vi "メイン.vi"() -> (2 "測定周期/ms":dbl, 3 "値転記用配列":T2[](array[typedef]))   [LabVIEW 2021] (continued)
                            n1019 = call-poly <vilib>:"Read Key.vi"("section"=w2857, "error in (no error)"=w2856, "key"=w2853, "refnum"=w2859) -> ("error out"=w2855:errorcluster, "value"=w2854:i32, "refnum out"=w2858:T10)  [unwired: 4 in, 1 out]
                            n1020 = Bundle By Name(cluster=w2851, "ポートNo."=w2854) -> (w2852:T2)
                          }
                          frame 4 {
                            n1021 = call-poly <vilib>:"Read Key.vi"("section"=w2866, "error in (no error)"=w2865, "key"=w2862, "refnum"=w2868) -> ("error out"=w2864:errorcluster, "value"=w2863:i32, "refnum out"=w2867:T10)  [unwired: 4 in, 1 out]
                            n1022 = Bundle By Name(cluster=w2860, "測定モード"=w2863) -> (w2861:T2)
                          }
                          frame 5 {
                            n1023 = call-poly <vilib>:"Read Key.vi"("section"=w2875, "error in (no error)"=w2874, "key"=w2871, "refnum"=w2877) -> ("error out"=w2873:errorcluster, "value"=w2872:string, "refnum out"=w2876:T10)  [unwired: 4 in, 1 out]
                            n1024 = Bundle By Name(cluster=w2870, "規格単位"=w2872) -> (w2869:T2)
                          }
                          frame 6 {
                            n1025 = call-poly <vilib>:"Read Key.vi"("section"=w2884, "error in (no error)"=w2883, "key"=w2880, "refnum"=w2886) -> ("error out"=w2882:errorcluster, "value"=w2881:string, "refnum out"=w2885:T10)  [unwired: 4 in, 1 out]
                            n1026 = Bundle By Name(cluster=w2879, "品質チェック項目"=w2881) -> (w2878:T2)
                          }
                          frame 7 {
                            n1027 = call-poly <vilib>:"Read Key.vi"("section"=w2893, "error in (no error)"=w2892, "key"=w2889, "refnum"=w2895) -> ("error out"=w2891:errorcluster, "value"=w2890:i32, "refnum out"=w2894:T10)  [unwired: 4 in, 1 out]
                            n1028 = Bundle By Name(cluster=w2888, "測定周期"=w2890) -> (w2887:T2)
                          }
                          frame 8 {
                            n1029 = call-poly <vilib>:"Read Key.vi"("section"=w2902, "error in (no error)"=w2901, "key"=w2898, "refnum"=w2904) -> ("error out"=w2900:errorcluster, "value"=w2899:string, "refnum out"=w2903:T10)  [unwired: 4 in, 1 out]
                            n1030 = Bundle By Name(cluster=w2896, "実測値MAX"=w2899) -> (w2897:T2)
                          }
                          frame 9 {
                            n1031 = call-poly <vilib>:"Read Key.vi"("section"=w2911, "error in (no error)"=w2910, "key"=w2907, "refnum"=w2913) -> ("error out"=w2909:errorcluster, "value"=w2908:string, "refnum out"=w2912:T10)  [unwired: 4 in, 1 out]
                            n1032 = Bundle By Name(cluster=w2905, "実測値MIN"=w2908) -> (w2906:T2)
                          }
                          frame 10 {
                            n1033 = call-poly <vilib>:"Read Key.vi"("section"=w2920, "error in (no error)"=w2919, "key"=w2916, "refnum"=w2922) -> ("error out"=w2918:errorcluster, "value"=w2917:string, "refnum out"=w2921:T10)  [unwired: 4 in, 1 out]
                            n1034 = Bundle By Name(cluster=w2914, "実測値(MAX)"=w2917) -> (w2915:T2)
                          }
                          frame 11 {
                            n1035 = call-poly <vilib>:"Read Key.vi"("section"=w2929, "error in (no error)"=w2928, "key"=w2925, "refnum"=w2931) -> ("error out"=w2927:errorcluster, "value"=w2926:string, "refnum out"=w2930:T10)  [unwired: 4 in, 1 out]
                            n1036 = Bundle By Name(cluster=w2923, "実測値(MIN)"=w2926) -> (w2924:T2)
                          }
                          frame 12 {
                            n1037 = call-poly <vilib>:"Read Key.vi"("section"=w2938, "error in (no error)"=w2937, "key"=w2934, "refnum"=w2940) -> ("error out"=w2936:errorcluster, "value"=w2935:bool, "refnum out"=w2939:T10)  [unwired: 4 in, 1 out]
                            n1038 = Bundle By Name(cluster=w2932, "測定画面表示ボタン"=w2935) -> (w2933:T2)
                          }
                          frame 13 {
                            n1039 = call-poly <vilib>:"Read Key.vi"("section"=w2947, "error in (no error)"=w2946, "key"=w2943, "refnum"=w2949) -> ("error out"=w2945:errorcluster, "value"=w2944:string, "refnum out"=w2948:T10)  [unwired: 4 in, 1 out]
                            n1040 = Bundle By Name(cluster=w2941, "ゲージポートNo"=w2944) -> (w2942:T2)
                          }
                        }
                        n1041 = local write "メイン設定_設定 12"(w2817) -> ()
                      }
                      n1042 = local read "メインON/OFF_\n設定 12"() -> (w2801:T1)
                      n1043 = call-poly <vilib>:"Read Key.vi"("section"=w2790, "error in (no error)"=w2808, "key"="使用ON/OFF", "refnum"=w2809) -> ("error out"=w2793:errorcluster, "value"=w2799:bool, "refnum out"=w2794:T10)  [unwired: 4 in, 1 out]
                      n1044 = Bundle By Name(cluster=w2801, "使用ON/OFF"=w2799) -> (w2802:T1)
                      n1045 = local write "メインON/OFF_\n設定 12"(w2802) -> ()
                      n1046 = local read "CSV項目名 12"() -> (w2798:T3)
                      n1047 = call-poly <vilib>:"Read Key.vi"("section"=w2790, "error in (no error)"=w2793, "key"="CSVヘッダー名", "refnum"=w2794) -> ("error out"=w2791:errorcluster, "value"=w2796:string, "refnum out"=w2792:T10)  [unwired: 4 in, 1 out]
                      n1048 = Bundle By Name(cluster=w2798, "CSV項目名"=w2796) -> (w2797:T3)
                      n1049 = local write "CSV項目名 12"(w2797) -> ()
                    }
                    frame #1 {
                      # "csvヘッダー項目作成"
                      # "⑮"
                      # "⑤"
                      n1050 = local read "CSV項目名 12"() -> (w2954:T3)
                      n1051 = Unbundle By Name(w2954) -> ("CSV項目名"=w2951:string)
                      n1052 = local read "メイン設定_設定 12"() -> (w2955:T2)
                      n1053 = Unbundle By Name(w2955) -> ("測定モード"=w2950:u16)
                      n1054 = case shown="0, デフォルト" w2950 {
                        tunnel: ["単発測定" _ "多点測定"] -> w2958
                        tunnel: [FALSE TRUE FALSE] -> w2957
                        tunnel: [TRUE FALSE TRUE] -> w2956
                        frame 0, Default {
                        }
                        frame 1 {
                        }
                        frame 2 {
                        }
                      }
                      n1055 = case shown="1" w2950 {
                        tunnel: w2951 -> [w2964 w2976 w2985]
                        tunnel: [w2962 w2974 w2987] -> w2953
                        tunnel: [w2961 w2973 w2986] -> w2952
                        frame 1 {
                          n1056 = Empty String/Path?(string/path=w2964) -> (empty?=w2963:bool)
                          n1057 = case shown="FALSE" w2963 {
                            tunnel: w2964 -> [w2970 _]
                            tunnel: w2964 -> [w2969 _]
                            tunnel: [w2966 ""] -> w2962
                            tunnel: [w2965 ""] -> w2961
                            frame False {
                              n1058 = Concatenate Strings(w2970, "_max") -> (w2966:string)
                              n1059 = Concatenate Strings(w2969, "_min") -> (w2965:string)
                            }
                            frame True {
                            }
                          }
                        }
                        frame 2 {
                          n1060 = Empty String/Path?(string/path=w2976) -> (empty?=w2975:bool)
                          n1061 = case shown="FALSE" w2975 {
                            tunnel: w2976 -> [w2982 _]
                            tunnel: w2976 -> [w2981 _]
                            tunnel: [w2978 ""] -> w2974
                            tunnel: [w2977 ""] -> w2973
                            frame False {
                              n1062 = Concatenate Strings(w2982, "_max") -> (w2978:string)
                              n1063 = Concatenate Strings(w2981, "_min") -> (w2977:string)
                            }
                            frame True {
                            }
                          }
                        }
                        frame 0, Default {
                          n1064 = Empty String/Path?(string/path=w2985) -> (empty?=w2988:bool)
                          n1065 = case shown="FALSE" w2988 {
                            tunnel: w2985 -> [w2992 _]
                            tunnel: [w2990 ""] -> w2987
                            tunnel: ["" ""] -> w2986
                            frame False {
                              n1066 = Concatenate Strings(w2992, "_value") -> (w2990:string)
                            }
                            frame True {
                            }
                          }
                        }
                      }
                      n1067 = property on="メイン測定ボタン_単発 12" class="Bool (指定)"("BoolText.Text"=w2958) -> ()  [unwired: 2 in, 2 out]
                      n1068 = local write "csv入力項目min 12"(w2952) -> ()
                      n1069 = local write "csv入力項目max 12"(w2953) -> ()
                      n1070 = property on="メイン測定ボタン_連続 12" class="Bool (指定)"("Visible"=w2957) -> ()  [unwired: 2 in, 2 out]
                      n1071 = property on="メイン測定ボタン_単発 12" class="Bool (指定)"("Visible"=w2956) -> ()  [unwired: 2 in, 2 out]
                    }
                    frame #2 {
                      # "⑯"
                      # "⑨"
                      # "⑧"
                      # "⑦"
                      # "⑥"
                      n1072 = local read "メインON/OFF_\n設定 12"() -> (w3006:T1)
                      n1073 = local write "メインON/OFF_\n保存確認 12"(w3006) -> ()
                      n1074 = local read "メイン設定_設定 12"() -> (w3004:T2)
                      n1075 = Unbundle By Name(w3004) -> ("測定画面表示ボタン"=w3003:bool)
                      n1076 = case shown="FALSE" w3003 {
                        tunnel: [w3009 TRUE] -> w3005
                        frame False {
                          w3009 = FALSE
                          n1077 = property on="メイン測定ボタン_単発 12" class="Bool (指定)"("Visible"=w3009) -> ()  [unwired: 2 in, 2 out]
                          n1078 = property on="メイン測定ボタン_連続 12" class="Bool (指定)"("Visible"=w3009) -> ()  [unwired: 2 in, 2 out]
                        }
                        frame True {
                        }
                      }
                      n1079 = local write "メインON/OFF_制御器 12"(w3006) -> ()
                      n1080 = property on="メインON/OFF_制御器 12" class="Clust (指定)"("Visible"=w3005) -> ()  [unwired: 2 in, 2 out]
                      n1081 = property on="メイン設定No_設定 12" class="Clust (指定)"("Visible"=w3005) -> ()  [unwired: 2 in, 2 out]
                      n1082 = property on="メイン設定_設定 12" class="Clust (指定)"("Visible"=w3005) -> ()  [unwired: 2 in, 2 out]
                      n1083 = property on="キャンセルボタン 12" class="Bool (指定)"("Visible"=w3005) -> ()  [unwired: 2 in, 2 out]
                    }
                  }
                  n1084 = Replace Array Subset(array=w2785, new element=w2777, index=11) -> (w2784:T2[])
                }
              }
              n1085 = property on="値転記用配列" class="Arr (指定)"("Value"=w70) -> ()  [unwired: 2 in, 2 out]
              n1086 = call <vilib>:"Close Config Data.vi"("error in (no error)"=w72, "refnum"=w73) -> ("error out"=→"setup.iniエラーout":errorcluster)  [unwired: 1 in, 8 out]
            }
          }
          frame #1 {
            # "csv作成表　を置換処理させる為の初期化"
            # "csv作成表_csv書込み　を置換処理させる為の初期化"
            n1087 = for {
              N: 3 -> [_]
              tunnel: [w3019] -> w3011 mode=indexing
              i -> [w3020]
              n1088 = case shown="0, デフォルト" w3020 {
                tunnel: [w3021 w3051 w3053] -> w3019
                frame 0, Default {
                  # "CSVマスターインポートファイル名を作成しA1セルに表示"
                  n1089 = local read "CSV保存名"() -> (w3022:string)
                  n1090 = Concatenate Strings("Sokutei_", w3022) -> (w3023:string)
                  n1091 = Build Array(w3023) -> (w3021:string[])
                }
                frame 1 {
                  n1092 = local read "csv入力項目max 11"() -> (w3028:string)
                  n1093 = local read "csv入力項目max 1"() -> (w3048:string)
                  n1094 = local read "csv入力項目max 3"() -> (w3044:string)
                  n1095 = local read "csv入力項目max 5"() -> (w3040:string)
                  n1096 = local read "csv入力項目max 7"() -> (w3036:string)
                  n1097 = local read "csv入力項目max 9"() -> (w3032:string)
                  n1098 = local read "csv入力項目min 11"() -> (w3027:string)
                  n1099 = local read "csv入力項目min 1"() -> (w3047:string)
                  n1100 = local read "csv入力項目min 3"() -> (w3043:string)
                  n1101 = local read "csv入力項目min 5"() -> (w3039:string)
                  n1102 = local read "csv入力項目min 7"() -> (w3035:string)
                  n1103 = local read "csv入力項目min 9"() -> (w3031:string)
                  n1104 = local read "csv入力項目max 2"() -> (w3046:string)
                  n1105 = local read "csv入力項目max 4"() -> (w3042:string)
                  n1106 = local read "csv入力項目max 6"() -> (w3038:string)
                  n1107 = local read "csv入力項目max 8"() -> (w3034:string)
                  n1108 = local read "csv入力項目max 10"() -> (w3030:string)
                  n1109 = local read "csv入力項目max 12"() -> (w3026:string)
                  n1110 = local read "csv入力項目min 2"() -> (w3045:string)
                  n1111 = local read "csv入力項目min 4"() -> (w3041:string)
                  n1112 = local read "csv入力項目min 6"() -> (w3037:string)
                  n1113 = local read "csv入力項目min 8"() -> (w3033:string)
                  n1114 = local read "csv入力項目min 10"() -> (w3029:string)
                  n1115 = local read "csv入力項目min 12"() -> (w3025:string)
                  n1116 = Build Array("Date", "Time", w3048, w3047, w3046, w3045, w3044, w3043, w3042, w3041, w3040, w3039, w3038, w3037, w3036, w3035, w3034, w3033, w3032, w3031, w3030, w3029, w3028, w3027, w3026, w3025) -> (w3051:string[])
                }
                frame 2 {
                  # "csv作成表の3行目の初期化\n配列置換する為の処理　\n並列処理は仮\nループ使用で考え直す"
                  n1117 = call <vilib>:"Space Constant.vi"() -> ("String"=w3052:string)
                  n1118 = Build Array(w3052, w3052, w3052, w3052, w3052, w3052, w3052, w3052, w3052, w3052, w3052, w3052, w3052, w3052, w3052, w3052, w3052, w3052, w3052, w3052, w3052, w3052, w3052, w3052, w3052, w3052, w3052, w3052, w3052, w3052, w3052, w3052, w3052, w3052, w3052, w3052, w3052, w3052, w3052, w3052, w3052, w3052, w3052, w3052, w3052) -> (w3053:string[])
                }
              }
            }
            n1119 = for {
              N: 66 -> [_]
              i -> [w3017]
              n1120 = local read "csv作成表_csv書込"() -> (w3018:string[][])
              n1121 = Insert Into Array(array=w3018, index (col)=w3017, new element=string[][] [["  ", " ", " "], ["  ", "", ""], ["  ", "", ""]]) -> (w3015:string[][])  [unwired: 1 in]
              n1122 = local write "csv作成表_csv書込_リセット用"(w3015) -> ()
              n1123 = local write "csv作成表_csv書込"(w3015) -> ()
            }
            n1124 = local write "csv作成表_リセット用"(w3011) -> ()
            n1125 = local write "csv作成表"(w3011) -> ()
          }
        }
      }
      frame "ON/OFF1" {
        # "①"
        # "②"
        # "他複製時に変更する項目\n①②\nローカル変数"
        # "メイン画面で作業者が測定値の転記のON/OFFを設定する"
        n1126 = local read "メインON/OFF_制御器 1"() -> (w3054:T1)
        n1127 = local write "メインON/OFF_\n設定 1"(w3054) -> ()
      }
      frame "ON/OFF2" {
        # "①"
        # "②"
        # "他複製時に変更する項目\n①②\nローカル変数"
        # "メイン画面で作業者が測定値の転記のON/OFFを設定する"
        n1128 = local read "メインON/OFF_制御器 2"() -> (w3056:T1)
        n1129 = local write "メインON/OFF_\n設定 2"(w3056) -> ()
      }
      frame "ON/OFF3" {
        # "①"
        # "②"
        # "他複製時に変更する項目\n①②\nローカル変数"
        # "メイン画面で作業者が測定値の転記のON/OFFを設定する"
        n1130 = local read "メインON/OFF_制御器 3"() -> (w3058:T1)
        n1131 = local write "メインON/OFF_\n設定 3"(w3058) -> ()
      }
      frame "ON/OFF4" {
        # "①"
        # "②"
        # "他複製時に変更する項目\n①②\nローカル変数"
        # "メイン画面で作業者が測定値の転記のON/OFFを設定する"
        n1132 = local read "メインON/OFF_制御器 4"() -> (w3060:T1)
        n1133 = local write "メインON/OFF_\n設定 4"(w3060) -> ()
      }
      frame "ON/OFF5" {
        # "①"
        # "②"
        # "他複製時に変更する項目\n①②\nローカル変数"
        # "メイン画面で作業者が測定値の転記のON/OFFを設定する"
        n1134 = local read "メインON/OFF_制御器 5"() -> (w3062:T1)
        n1135 = local write "メインON/OFF_\n設定 5"(w3062) -> ()
      }
      frame "ON/OFF6" {
        # "①"
        # "②"
        # "他複製時に変更する項目\n①②\nローカル変数"
        # "メイン画面で作業者が測定値の転記のON/OFFを設定する"
        n1136 = local read "メインON/OFF_制御器 6"() -> (w3064:T1)
        n1137 = local write "メインON/OFF_\n設定 6"(w3064) -> ()
      }
      frame "ON/OFF7" {
        # "①"
        # "②"
        # "他複製時に変更する項目\n①②\nローカル変数"
        # "メイン画面で作業者が測定値の転記のON/OFFを設定する"
        n1138 = local read "メインON/OFF_制御器 7"() -> (w3066:T1)
        n1139 = local write "メインON/OFF_\n設定 7"(w3066) -> ()
      }
      frame "ON/OFF8" {
        # "①"
        # "②"
        # "他複製時に変更する項目\n①②\nローカル変数"
        # "メイン画面で作業者が測定値の転記のON/OFFを設定する"
        n1140 = local read "メインON/OFF_制御器 8"() -> (w3068:T1)
        n1141 = local write "メインON/OFF_\n設定 8"(w3068) -> ()
      }
      frame "ON/OFF9" {
        # "①"
        # "②"
        # "他複製時に変更する項目\n①②\nローカル変数"
        # "メイン画面で作業者が測定値の転記のON/OFFを設定する"
        n1142 = local read "メインON/OFF_制御器 9"() -> (w3070:T1)
        n1143 = local write "メインON/OFF_\n設定 9"(w3070) -> ()
      }
      frame "ON/OFF10" {
        # "①"
        # "②"
        # "他複製時に変更する項目\n①②\nローカル変数"
        # "メイン画面で作業者が測定値の転記のON/OFFを設定する"
        n1144 = local read "メインON/OFF_制御器 10"() -> (w3072:T1)
        n1145 = local write "メインON/OFF_\n設定 10"(w3072) -> ()
      }
      frame "ON/OFF11" {
        # "①"
        # "②"
        # "他複製時に変更する項目\n①②\nローカル変数"
        # "メイン画面で作業者が測定値の転記のON/OFFを設定する"
        n1146 = local read "メインON/OFF_制御器 11"() -> (w3074:T1)
        n1147 = local write "メインON/OFF_\n設定 11"(w3074) -> ()
      }
      frame "ON/OFF12" {
        # "①"
        # "②"
        # "他複製時に変更する項目\n①②\nローカル変数"
        # "メイン画面で作業者が測定値の転記のON/OFFを設定する"
        n1148 = local read "メインON/OFF_制御器 12"() -> (w3076:T1)
        n1149 = local write "メインON/OFF_\n設定 12"(w3076) -> ()
      }
      frame "TOPページへ" {
        w3078 = TRUE
        # "メインviを閉じるのみの動作"
        n1150 = flat-sequence {
          tunnel: w3078 -> [w3080]
          tunnel: [w3081] -> w3079
          tunnel: w3078 -> [w3081]
          frame #0 {
            n1151 = global write "VISA停止_G.vi" "VISA停止_\nグローバル"(w3080) -> ()
          }
          frame #1 {
          }
        }
      }
      frame "保存せず" {
        w3087 = T9 {"Horizontal"=-51, "Vertical"=0} ("座標 1")
        # "csv作成表の初期化"
        # "赤枠の初期化"
        # "②"
        # "①"
        # "全ての項目に適応の為、このケースでのみで処理"
        # "①測定値を空にする処理\n複製した項目を追加する必要がある\n②測定新値リセットをFalseにする\nⅠ.初期設定⑥\nと同じなので、どちらか項目を追加したらコピーする"
        n1152 = for {
          N: 32 -> [_]
          i -> [w3106]
          n1153 = case shown="0, デフォルト" w3106 {
            frame 0, Default {
              w3109 = ""
              n1154 = local read "メイン設定_設定 1"() -> (w3108:T2)
              n1155 = Bundle By Name(cluster=w3108, "実測値(MAX)"=w3109, "実測値(MIN)"=w3109) -> (w3107:T2)
              n1156 = local write "メイン設定_設定 1"(w3107) -> ()
            }
            frame 1 {
              w3112 = ""
              n1157 = local read "メイン設定_設定 2"() -> (w3111:T2)
              n1158 = Bundle By Name(cluster=w3111, "実測値(MAX)"=w3112, "実測値(MIN)"=w3112) -> (w3110:T2)
              n1159 = local write "メイン設定_設定 2"(w3110) -> ()
            }
            frame 2 {
              w3115 = ""
              n1160 = local read "メイン設定_設定 3"() -> (w3114:T2)
              n1161 = Bundle By Name(cluster=w3114, "実測値(MAX)"=w3115, "実測値(MIN)"=w3115) -> (w3113:T2)
              n1162 = local write "メイン設定_設定 3"(w3113) -> ()
            }
            frame 3 {
              w3118 = ""
              n1163 = local read "メイン設定_設定 4"() -> (w3117:T2)
              n1164 = Bundle By Name(cluster=w3117, "実測値(MAX)"=w3118, "実測値(MIN)"=w3118) -> (w3116:T2)
              n1165 = local write "メイン設定_設定 4"(w3116) -> ()
            }
            frame 4 {
              w3121 = ""
              n1166 = local read "メイン設定_設定 5"() -> (w3120:T2)
              n1167 = Bundle By Name(cluster=w3120, "実測値(MAX)"=w3121, "実測値(MIN)"=w3121) -> (w3119:T2)
              n1168 = local write "メイン設定_設定 5"(w3119) -> ()
            }
            frame 5 {
              w3124 = ""
              n1169 = local read "メイン設定_設定 6"() -> (w3123:T2)
              n1170 = Bundle By Name(cluster=w3123, "実測値(MAX)"=w3124, "実測値(MIN)"=w3124) -> (w3122:T2)
              n1171 = local write "メイン設定_設定 6"(w3122) -> ()
            }
            frame 6 {
              w3127 = ""
              n1172 = local read "メイン設定_設定 7"() -> (w3126:T2)
              n1173 = Bundle By Name(cluster=w3126, "実測値(MAX)"=w3127, "実測値(MIN)"=w3127) -> (w3125:T2)
              n1174 = local write "メイン設定_設定 7"(w3125) -> ()
            }
            frame 7 {
              w3130 = ""
              n1175 = local read "メイン設定_設定 8"() -> (w3129:T2)
              n1176 = Bundle By Name(cluster=w3129, "実測値(MAX)"=w3130, "実測値(MIN)"=w3130) -> (w3128:T2)
              n1177 = local write "メイン設定_設定 8"(w3128) -> ()
            }
            frame 8 {
              w3133 = ""
              n1178 = local read "メイン設定_設定 9"() -> (w3132:T2)
              n1179 = Bundle By Name(cluster=w3132, "実測値(MAX)"=w3133, "実測値(MIN)"=w3133) -> (w3131:T2)
              n1180 = local write "メイン設定_設定 9"(w3131) -> ()
            }
            frame 9 {
              w3136 = ""
              n1181 = local read "メイン設定_設定 10"() -> (w3135:T2)
              n1182 = Bundle By Name(cluster=w3135, "実測値(MAX)"=w3136, "実測値(MIN)"=w3136) -> (w3134:T2)
              n1183 = local write "メイン設定_設定 10"(w3134) -> ()
            }
            frame 10 {
              w3139 = ""
              n1184 = local read "メイン設定_設定 11"() -> (w3138:T2)
              n1185 = Bundle By Name(cluster=w3138, "実測値(MAX)"=w3139, "実測値(MIN)"=w3139) -> (w3137:T2)
              n1186 = local write "メイン設定_設定 11"(w3137) -> ()
            }
            frame 11 {
              w3142 = ""
              n1187 = local read "メイン設定_設定 12"() -> (w3141:T2)
              n1188 = Bundle By Name(cluster=w3141, "実測値(MAX)"=w3142, "実測値(MIN)"=w3142) -> (w3140:T2)
              n1189 = local write "メイン設定_設定 12"(w3140) -> ()
            }
          }
        }
        n1190 = for {
          N: 32 -> [_]
          tunnel: FALSE -> [w3092]
          i -> [w3093]
          n1191 = case shown="0, デフォルト" w3093 {
            tunnel: w3092 -> [w3094 w3095 w3096 w3097 w3098 w3099 w3100 w3101 w3102 w3103 w3104 w3105]
            frame 0, Default {
              n1192 = local write "測定新値\nリセット用 1"(w3094) -> ()
              n1193 = local write "測定旧値 1"(w3094) -> ()
            }
            frame 1 {
              n1194 = local write "測定新値\nリセット用 2"(w3095) -> ()
              n1195 = local write "測定旧値 2"(w3095) -> ()
            }
            frame 2 {
              n1196 = local write "測定新値\nリセット用 3"(w3096) -> ()
              n1197 = local write "測定旧値 3"(w3096) -> ()
            }
            frame 3 {
              n1198 = local write "測定新値\nリセット用 4"(w3097) -> ()
              n1199 = local write "測定旧値 4"(w3097) -> ()
            }
            frame 4 {
              n1200 = local write "測定新値\nリセット用 5"(w3098) -> ()
              n1201 = local write "測定旧値 5"(w3098) -> ()
            }
            frame 5 {
              n1202 = local write "測定新値\nリセット用 6"(w3099) -> ()
              n1203 = local write "測定旧値 6"(w3099) -> ()
            }
            frame 6 {
              n1204 = local write "測定新値\nリセット用 7"(w3100) -> ()
              n1205 = local write "測定旧値 7"(w3100) -> ()
            }
            frame 7 {
              n1206 = local write "測定新値\nリセット用 8"(w3101) -> ()
              n1207 = local write "測定旧値 8"(w3101) -> ()
            }
            frame 8 {
              n1208 = local write "測定新値\nリセット用 9"(w3102) -> ()
              n1209 = local write "測定旧値 9"(w3102) -> ()
            }
            frame 9 {
              n1210 = local write "測定新値\nリセット用 10"(w3103) -> ()
              n1211 = local write "測定旧値 10"(w3103) -> ()
            }
            frame 10 {
              n1212 = local write "測定新値\nリセット用 11"(w3104) -> ()
              n1213 = local write "測定旧値 11"(w3104) -> ()
            }
            frame 11 {
              n1214 = local write "測定新値\nリセット用 12"(w3105) -> ()
              n1215 = local write "測定旧値 12"(w3105) -> ()
            }
          }
        }
        n1216 = control-ref of="このVI"() -> (w3085:refnum<vi>)
        n1217 = property on="ペーン 2" class="Pane"("Origin"=w3087) -> ()  [unwired: 2 in, 2 out]
        n1218 = control-ref of="このVI"() -> (w3086:refnum<vi>)
        n1219 = Unbundle(w3087) -> ("Vertical"=w3084:i16)  [unwired: 1 out]
        n1220 = Unbundle(w3087) -> ()  [unwired: 2 out]
        n1221 = property on="ペーン 2" class="Pane"("Origin"=w3087) -> ()  [unwired: 2 in, 2 out]
        n1222 = call "メイン_装飾移動サブ.vi"("Y軸座標入力"=w3084, "VI入力"=w3085) -> ()  [unwired: 10 in]
        n1223 = call "メイン_装飾枠移動サブ.vi"("VI入力"=w3086) -> ()  [unwired: 11 in]
        n1224 = local read "csv作成表_csv書込_リセット用"() -> (w3082:string[][])
        n1225 = local read "csv作成表_リセット用"() -> (w3083:string[][])
        n1226 = local write "csv作成表_csv書込"(w3082) -> ()
        n1227 = local write "csv作成表"(w3083) -> ()
      }
      frame "保存して終了" {
        w3146 = T9 {"Horizontal"=-51, "Vertical"=0} ("座標 1")
        # "赤枠の初期化"
        # "項目複製した場合\n①値が書き込まれているか確認するケース\n対象項目を複製し追加する\n②ダイアログ表示有無\n何もしなくてＯＫ\n③測定値の処理\n対象項目を複製し追加する\nTrueとFalseともに\n④CSV書き込み\n何もしなくてOK"
        # "※TRUEならﾒｲﾝ設定_設定　に空を入れる\nFalseなら元に戻す\n設定毎に\n書き込みはこの後におこなう必要がある"
        # "測定値の値が空か？　＝＞　空じゃない　＝＞　品番_日時_秒.csv名で指定フォルダに保存\n　　　　　　　　　　　　空だったら　＝＞　保存する　＝＞　品番_日時_秒.csv名で指定フォルダに保存\n　　　　　　　　　　　　　　　　　＝＞　キャンセル　＝＞　iniファイルを呼び出す"
        # "保存して次の測定への処理"
        n1228 = flat-sequence {
          frame #0 {
            n1229 = local write "保存ブール"(FALSE) -> ()
          }
          frame #1 {
            # "※ここは32回繰り返し、入力されているかかくにんする必要がある"
            # "測定値の値がMAXや値に書き込まれているかをboolする"
            n1230 = for {
              N: 32 -> [_]
              i -> [w3150]
              # "①"
              n1231 = case shown="11" w3150 {
                frame 0, Default {
                  n1232 = local read "メインON/OFF_\n保存確認 1"() -> (w3152:T1)
                  n1233 = Unbundle By Name(w3152) -> ("使用ON/OFF"=w3151:bool)
                  n1234 = case shown="TRUE" w3151 {
                    frame False {
                    }
                    frame True {
                      n1235 = local read "メイン設定_設定 1"() -> (w3154:T2)
                      n1236 = for {
                        N: 1 -> [_]
                        tunnel: w3154 -> [w3157]
                        # "空=TRUEだったらダイアログを出す"
                        n1237 = Unbundle By Name(w3157) -> ("実測値(MAX)"=w3155:string)
                        n1238 = Empty String/Path?(string/path=w3155) -> (empty?=w3156:bool)
                        n1239 = case shown="TRUE" w3156 {
                          frame False {
                          }
                          frame True {
                            n1240 = local write "保存ブール"(TRUE) -> ()
                          }
                        }
                      }
                    }
                  }
                }
                frame 1 {
                  n1241 = local read "メインON/OFF_\n保存確認 2"() -> (w3160:T1)
                  n1242 = Unbundle By Name(w3160) -> ("使用ON/OFF"=w3159:bool)
                  n1243 = case shown="TRUE" w3159 {
                    frame False {
                    }
                    frame True {
                      n1244 = local read "メイン設定_設定 2"() -> (w3162:T2)
                      n1245 = for {
                        N: 1 -> [_]
                        tunnel: w3162 -> [w3165]
                        # "空=TRUEだったらダイアログを出す"
                        n1246 = Unbundle By Name(w3165) -> ("実測値(MAX)"=w3163:string)
                        n1247 = Empty String/Path?(string/path=w3163) -> (empty?=w3164:bool)
                        n1248 = case shown="TRUE" w3164 {
                          frame False {
                          }
                          frame True {
                            n1249 = local write "保存ブール"(TRUE) -> ()
                          }
                        }
                      }
                    }
                  }
                }
                frame 2 {
                  n1250 = local read "メインON/OFF_\n保存確認 3"() -> (w3168:T1)
                  n1251 = Unbundle By Name(w3168) -> ("使用ON/OFF"=w3167:bool)
                  n1252 = case shown="TRUE" w3167 {
                    frame False {
                    }
                    frame True {
                      n1253 = local read "メイン設定_設定 3"() -> (w3170:T2)
                      n1254 = for {
                        N: 1 -> [_]
                        tunnel: w3170 -> [w3173]
                        # "空=TRUEだったらダイアログを出す"
                        n1255 = Unbundle By Name(w3173) -> ("実測値(MAX)"=w3171:string)
                        n1256 = Empty String/Path?(string/path=w3171) -> (empty?=w3172:bool)
                        n1257 = case shown="TRUE" w3172 {
                          frame False {
                          }
                          frame True {
                            n1258 = local write "保存ブール"(TRUE) -> ()
                          }
                        }
                      }
                    }
                  }
                }
                frame 3 {
                  n1259 = local read "メインON/OFF_\n保存確認 4"() -> (w3176:T1)
                  n1260 = Unbundle By Name(w3176) -> ("使用ON/OFF"=w3175:bool)
                  n1261 = case shown="TRUE" w3175 {
                    frame False {
                    }
                    frame True {
                      n1262 = local read "メイン設定_設定 4"() -> (w3178:T2)
                      n1263 = for {
                        N: 1 -> [_]
                        tunnel: w3178 -> [w3181]
                        # "空=TRUEだったらダイアログを出す"
                        n1264 = Unbundle By Name(w3181) -> ("実測値(MAX)"=w3179:string)
                        n1265 = Empty String/Path?(string/path=w3179) -> (empty?=w3180:bool)
                        n1266 = case shown="TRUE" w3180 {
                          frame False {
                          }
                          frame True {
                            n1267 = local write "保存ブール"(TRUE) -> ()
                          }
                        }
                      }
                    }
                  }
                }
                frame 4 {
                  n1268 = local read "メインON/OFF_\n保存確認 5"() -> (w3184:T1)
                  n1269 = Unbundle By Name(w3184) -> ("使用ON/OFF"=w3183:bool)
                  n1270 = case shown="TRUE" w3183 {
                    frame False {
                    }
                    frame True {
                      n1271 = local read "メイン設定_設定 5"() -> (w3186:T2)
                      n1272 = for {
                        N: 1 -> [_]
                        tunnel: w3186 -> [w3189]
                        # "空=TRUEだったらダイアログを出す"
                        n1273 = Unbundle By Name(w3189) -> ("実測値(MAX)"=w3187:string)
                        n1274 = Empty String/Path?(string/path=w3187) -> (empty?=w3188:bool)
                        n1275 = case shown="TRUE" w3188 {
                          frame False {
                          }
                          frame True {
                            n1276 = local write "保存ブール"(TRUE) -> ()
                          }
                        }
                      }
                    }
                  }
                }
                frame 5 {
                  n1277 = local read "メインON/OFF_\n保存確認 6"() -> (w3192:T1)
                  n1278 = Unbundle By Name(w3192) -> ("使用ON/OFF"=w3191:bool)
                  n1279 = case shown="TRUE" w3191 {
                    frame False {
                    }
                    frame True {
                      n1280 = local read "メイン設定_設定 6"() -> (w3194:T2)
                      n1281 = for {
                        N: 1 -> [_]
                        tunnel: w3194 -> [w3197]
                        # "空=TRUEだったらダイアログを出す"
                        n1282 = Unbundle By Name(w3197) -> ("実測値(MAX)"=w3195:string)
                        n1283 = Empty String/Path?(string/path=w3195) -> (empty?=w3196:bool)
                        n1284 = case shown="TRUE" w3196 {
                          frame False {
                          }
                          frame True {
                            n1285 = local write "保存ブール"(TRUE) -> ()
                          }
                        }
                      }
                    }
                  }
                }
                frame 6 {
                  n1286 = local read "メインON/OFF_\n保存確認 7"() -> (w3200:T1)
                  n1287 = Unbundle By Name(w3200) -> ("使用ON/OFF"=w3199:bool)
                  n1288 = case shown="TRUE" w3199 {
                    frame False {
                    }
                    frame True {
                      n1289 = local read "メイン設定_設定 7"() -> (w3202:T2)
                      n1290 = for {
                        N: 1 -> [_]
                        tunnel: w3202 -> [w3205]
                        # "空=TRUEだったらダイアログを出す"
                        n1291 = Unbundle By Name(w3205) -> ("実測値(MAX)"=w3203:string)
                        n1292 = Empty String/Path?(string/path=w3203) -> (empty?=w3204:bool)
                        n1293 = case shown="FALSE" w3204 {
                          frame False {
                          }
                          frame True {
                            n1294 = local write "保存ブール"(TRUE) -> ()
                          }
                        }
                      }
                    }
                  }
                }
                frame 7 {
                  n1295 = local read "メインON/OFF_\n保存確認 8"() -> (w3208:T1)
                  n1296 = Unbundle By Name(w3208) -> ("使用ON/OFF"=w3207:bool)
                  n1297 = case shown="TRUE" w3207 {
                    frame False {
                    }
                    frame True {
                      n1298 = local read "メイン設定_設定 8"() -> (w3210:T2)
                      n1299 = for {
                        N: 1 -> [_]
                        tunnel: w3210 -> [w3213]
                        # "空=TRUEだったらダイアログを出す"
                        n1300 = Unbundle By Name(w3213) -> ("実測値(MAX)"=w3211:string)
                        n1301 = Empty String/Path?(string/path=w3211) -> (empty?=w3212:bool)
                        n1302 = case shown="FALSE" w3212 {
                          frame False {
                          }
                          frame True {
                            n1303 = local write "保存ブール"(TRUE) -> ()
                          }
                        }
                      }
                    }
                  }
                }
                frame 8 {
                  n1304 = local read "メインON/OFF_\n保存確認 9"() -> (w3216:T1)
                  n1305 = Unbundle By Name(w3216) -> ("使用ON/OFF"=w3215:bool)
                  n1306 = case shown="TRUE" w3215 {
                    frame False {
                    }
                    frame True {
                      n1307 = local read "メイン設定_設定 9"() -> (w3218:T2)
                      n1308 = for {
                        N: 1 -> [_]
                        tunnel: w3218 -> [w3221]
                        # "空=TRUEだったらダイアログを出す"
                        n1309 = Unbundle By Name(w3221) -> ("実測値(MAX)"=w3219:string)
                        n1310 = Empty String/Path?(string/path=w3219) -> (empty?=w3220:bool)
                        n1311 = case shown="FALSE" w3220 {
                          frame False {
                          }
                          frame True {
                            n1312 = local write "保存ブール"(TRUE) -> ()
                          }
                        }
                      }
                    }
                  }
                }
                frame 9 {
                  n1313 = local read "メインON/OFF_\n保存確認 10"() -> (w3224:T1)
                  n1314 = Unbundle By Name(w3224) -> ("使用ON/OFF"=w3223:bool)
                  n1315 = case shown="TRUE" w3223 {
                    frame False {
                    }
                    frame True {
                      n1316 = local read "メイン設定_設定 10"() -> (w3226:T2)
                      n1317 = for {
                        N: 1 -> [_]
                        tunnel: w3226 -> [w3229]
                        # "空=TRUEだったらダイアログを出す"
                        n1318 = Unbundle By Name(w3229) -> ("実測値(MAX)"=w3227:string)
                        n1319 = Empty String/Path?(string/path=w3227) -> (empty?=w3228:bool)
                        n1320 = case shown="TRUE" w3228 {
                          frame False {
                          }
                          frame True {
                            n1321 = local write "保存ブール"(TRUE) -> ()
                          }
                        }
                      }
                    }
                  }
                }
                frame 10 {
                  n1322 = local read "メインON/OFF_\n保存確認 11"() -> (w3232:T1)
                  n1323 = Unbundle By Name(w3232) -> ("使用ON/OFF"=w3231:bool)
                  n1324 = case shown="TRUE" w3231 {
                    frame False {
                    }
                    frame True {
                      n1325 = local read "メイン設定_設定 11"() -> (w3234:T2)
                      n1326 = for {
                        N: 1 -> [_]
                        tunnel: w3234 -> [w3237]
                        # "空=TRUEだったらダイアログを出す"
                        n1327 = Unbundle By Name(w3237) -> ("実測値(MAX)"=w3235:string)
                        n1328 = Empty String/Path?(string/path=w3235) -> (empty?=w3236:bool)
                        n1329 = case shown="TRUE" w3236 {
                          frame False {
                          }
                          frame True {
                            n1330 = local write "保存ブール"(TRUE) -> ()
                          }
                        }
                      }
                    }
                  }
                }
                frame 11 {
                  n1331 = local read "メインON/OFF_\n保存確認 12"() -> (w3240:T1)
                  n1332 = Unbundle By Name(w3240) -> ("使用ON/OFF"=w3239:bool)
                  n1333 = case shown="TRUE" w3239 {
                    frame False {
                    }
                    frame True {
                      n1334 = local read "メイン設定_設定 12"() -> (w3242:T2)
                      n1335 = for {
                        N: 1 -> [_]
                        tunnel: w3242 -> [w3245]
                        # "空=TRUEだったらダイアログを出す"
                        n1336 = Unbundle By Name(w3245) -> ("実測値(MAX)"=w3243:string)
                        n1337 = Empty String/Path?(string/path=w3243) -> (empty?=w3244:bool)
                        n1338 = case shown="FALSE" w3244 {
                          frame False {
                          }
                          frame True {
                            n1339 = local write "保存ブール"(TRUE) -> ()
                          }
                        }
                      }
                    }
                  }
                }
              }
            }
          }
          frame #2 {
            # "②"
            n1340 = local read "保存ブール"() -> (w3247:bool)
            n1341 = case shown="TRUE" w3247 {
              frame False {
              }
              frame True {
                n1342 = Two Button Dialog(message="測定の値が入力されていません。そのまま保存しますか？", 1:"保存する", 2:"キャンセル") -> (T button?=w3248:bool)
                n1343 = local write "保存ブール"(w3248) -> ()
              }
            }
          }
          frame #3 {
            # "③"
            # "値の書き込みが\nFalseだったら実測値を空にする\nTrueだったら何もしない"
            n1344 = local read "保存ブール"() -> (w3261:bool)
            n1345 = case shown="FALSE" w3261 {
              tunnel: 32 -> [w3262 _]
              frame False {
                n1346 = for {
                  N: w3262 -> [_]
                  i -> [w3263]
                  n1347 = case shown="11" w3263 {
                    frame 0, Default {
                      w3266 = ""
                      n1348 = local read "メイン設定_設定 1"() -> (w3264:T2)
                      n1349 = Bundle By Name(cluster=w3264, "実測値(MAX)"=w3266, "実測値(MIN)"=w3266) -> (w3265:T2)
                      n1350 = local write "メイン設定_設定 1"(w3265) -> ()
                    }
                    frame 1 {
                      w3269 = ""
                      n1351 = local read "メイン設定_設定 2"() -> (w3267:T2)
                      n1352 = Bundle By Name(cluster=w3267, "実測値(MAX)"=w3269, "実測値(MIN)"=w3269) -> (w3268:T2)
                      n1353 = local write "メイン設定_設定 2"(w3268) -> ()
                    }
                    frame 2 {
                      w3272 = ""
                      n1354 = local read "メイン設定_設定 3"() -> (w3270:T2)
                      n1355 = Bundle By Name(cluster=w3270, "実測値(MAX)"=w3272, "実測値(MIN)"=w3272) -> (w3271:T2)
                      n1356 = local write "メイン設定_設定 3"(w3271) -> ()
                    }
                    frame 3 {
                      w3275 = ""
                      n1357 = local read "メイン設定_設定 4"() -> (w3273:T2)
                      n1358 = Bundle By Name(cluster=w3273, "実測値(MAX)"=w3275, "実測値(MIN)"=w3275) -> (w3274:T2)
                      n1359 = local write "メイン設定_設定 4"(w3274) -> ()
                    }
                    frame 4 {
                      w3278 = ""
                      n1360 = local read "メイン設定_設定 5"() -> (w3276:T2)
                      n1361 = Bundle By Name(cluster=w3276, "実測値(MAX)"=w3278, "実測値(MIN)"=w3278) -> (w3277:T2)
                      n1362 = local write "メイン設定_設定 5"(w3277) -> ()
                    }
                    frame 5 {
                      w3281 = ""
                      n1363 = local read "メイン設定_設定 6"() -> (w3279:T2)
                      n1364 = Bundle By Name(cluster=w3279, "実測値(MAX)"=w3281, "実測値(MIN)"=w3281) -> (w3280:T2)
                      n1365 = local write "メイン設定_設定 6"(w3280) -> ()
                    }
                    frame 6 {
                      w3284 = ""
                      n1366 = local read "メイン設定_設定 7"() -> (w3282:T2)
                      n1367 = Bundle By Name(cluster=w3282, "実測値(MAX)"=w3284, "実測値(MIN)"=w3284) -> (w3283:T2)
                      n1368 = local write "メイン設定_設定 7"(w3283) -> ()
                    }
                    frame 7 {
                      w3287 = ""
                      n1369 = local read "メイン設定_設定 8"() -> (w3285:T2)
                      n1370 = Bundle By Name(cluster=w3285, "実測値(MAX)"=w3287, "実測値(MIN)"=w3287) -> (w3286:T2)
                      n1371 = local write "メイン設定_設定 8"(w3286) -> ()
                    }
                    frame 8 {
                      w3290 = ""
                      n1372 = local read "メイン設定_設定 9"() -> (w3288:T2)
                      n1373 = Bundle By Name(cluster=w3288, "実測値(MAX)"=w3290, "実測値(MIN)"=w3290) -> (w3289:T2)
                      n1374 = local write "メイン設定_設定 9"(w3289) -> ()
                    }
                    frame 9 {
                      w3293 = ""
                      n1375 = local read "メイン設定_設定 10"() -> (w3291:T2)
                      n1376 = Bundle By Name(cluster=w3291, "実測値(MAX)"=w3293, "実測値(MIN)"=w3293) -> (w3292:T2)
                      n1377 = local write "メイン設定_設定 10"(w3292) -> ()
                    }
                    frame 10 {
                      w3296 = ""
                      n1378 = local read "メイン設定_設定 11"() -> (w3294:T2)
                      n1379 = Bundle By Name(cluster=w3294, "実測値(MAX)"=w3296, "実測値(MIN)"=w3296) -> (w3295:T2)
                      n1380 = local write "メイン設定_設定 11"(w3295) -> ()
                    }
                    frame 11 {
                      w3299 = ""
                      n1381 = local read "メイン設定_設定 12"() -> (w3297:T2)
                      n1382 = Bundle By Name(cluster=w3297, "実測値(MAX)"=w3299, "実測値(MIN)"=w3299) -> (w3298:T2)
                      n1383 = local write "メイン設定_設定 12"(w3298) -> ()
                    }
                  }
                }
              }
              frame True {
              }
            }
            n1384 = Format Date/Time String(time format string (%c)="\"%H:%M,%S\"" ("時間形式文字列 (%c)")) -> (date/time string=→"書込時間":string)  [unwired: 2 in]
            n1385 = Format Date/Time String(time format string (%c)="%Y/%m/%d" ("時間形式文字列 (%c)")) -> (date/time string=→"書込日付":string)  [unwired: 2 in]
            n1386 = Format Date/Time String(time format string (%c)="%H%M%S" ("時間形式文字列 (%c)")) -> (date/time string=→"書込CSV時間":string)  [unwired: 2 in]
            n1387 = Format Date/Time String(time format string (%c)="%Y%m%d" ("時間形式文字列 (%c)")) -> (date/time string=→"書込CSV日付":string)  [unwired: 2 in]
          }
          frame #4 {
            n1388 = local read "書込日付"() -> (w3300:string)
            n1389 = local read "csv作成表"() -> (w3304:string[][])
            n1390 = Replace Array Subset(array=w3304, new element=w3300, index (row)=2, index (col)=0) -> (w3303:string[][])
            n1391 = local write "csv作成表"(w3303) -> ()
          }
          frame #5 {
            n1392 = local read "書込時間"() -> (w3305:string)
            n1393 = local read "csv作成表"() -> (w3306:string[][])
            n1394 = Replace Array Subset(array=w3306, new element=w3305, index (row)=2, index (col)=1) -> (w3307:string[][])
            n1395 = local write "csv作成表"(w3307) -> ()
          }
          frame #6 {
            n1396 = for {
              N: 3 -> [_]
              i -> [w3311]
              n1397 = local read "csv作成表"() -> (w3312:string[][])
              n1398 = case shown="2" w3311 {
                tunnel: w3312 -> [w3316 w3325 w3343]
                tunnel: w3311 -> [w3315 w3324 w3342]
                tunnel: w3311 -> [w3314 w3323 w3341]
                frame 0, Default {
                  # "csv作成表の1行目をcsv書込へコピー\n加工必要ない為そのまま"
                  n1399 = Index Array(array=w3316, index (row)=w3315) -> (element=w3313:string[])  [unwired: 1 in]
                  n1400 = for {
                    tunnel: w3314 -> [w3319]
                    tunnel: w3313 -> [w3317] mode=indexing
                    i -> [w3318]
                    n1401 = local read "csv作成表_csv書込"() -> (w3321:string[][])
                    n1402 = Replace Array Subset(array=w3321, new element=w3317, index (row)=w3319, index (col)=w3318) -> (w3320:string[][])
                    n1403 = local write "csv作成表_csv書込"(w3320) -> ()
                  }
                }
                frame 1 {
                  # "csv作成表の2行目をcsv書込へコピー\n1行ずつコピーを行い、セルが空だったら行を詰める処理"
                  n1404 = Index Array(array=w3325, index (row)=w3324) -> (element=w3322:string[])  [unwired: 1 in]
                  n1405 = for {
                    tunnel: w3323 -> [w3326]
                    tunnel: w3322 -> [w3328] mode=indexing
                    i -> [w3327]
                    n1406 = Empty String/Path?(string/path=w3328) -> (empty?=w3329:bool)
                    n1407 = case shown="FALSE" w3329 {
                      tunnel: w3328 -> [w3336 _]
                      tunnel: w3327 -> [w3335 _]
                      tunnel: w3326 -> [w3332 _]
                      frame False {
                        # "ループの値-空白列カウント\nで空白列を削除して詰める"
                        n1408 = local read "csv作成表_csv書込"() -> (w3331:string[][])
                        n1409 = local read "空白列カウント"() -> (w3334:dbl)
                        n1410 = Subtract(x=w3335, y=w3334) -> (x-y=w3333:dbl)
                        n1411 = Replace Array Subset(array=w3331, new element=w3336, index (row)=w3332, index (col)=w3333) -> (w3330:string[][])
                        n1412 = local write "csv作成表_csv書込"(w3330) -> ()
                      }
                      frame True {
                        # "セルが空白だったらカウント1アップ"
                        n1413 = local read "空白列カウント"() -> (w3338:dbl)
                        n1414 = Add(x=w3338, y=1) -> (x+y=w3339:dbl)
                        n1415 = local write "空白列カウント"(w3339) -> ()
                      }
                    }
                  }
                }
                frame 2 {
                  # "csv作成表の3行目をcsv書込へコピー\n1行ずつコピーを行い、セルが空だったら行を詰める処理"
                  n1416 = Index Array(array=w3343, index (row)=w3342) -> (element=w3340:string[])  [unwired: 1 in]
                  n1417 = for {
                    tunnel: w3341 -> [w3344]
                    tunnel: w3340 -> [w3346] mode=indexing
                    i -> [w3345]
                    n1418 = Empty String/Path?(string/path=w3346) -> (empty?=w3347:bool)
                    n1419 = case shown="FALSE" w3347 {
                      tunnel: w3346 -> [w3354 _]
                      tunnel: w3345 -> [w3353 _]
                      tunnel: w3344 -> [w3350 _]
                      frame False {
                        # "ループの値-空白列カウント\nで空白列を削除して詰める"
                        n1420 = local read "csv作成表_csv書込"() -> (w3349:string[][])
                        n1421 = local read "空白列カウント 2"() -> (w3352:dbl)
                        n1422 = Subtract(x=w3353, y=w3352) -> (x-y=w3351:dbl)
                        n1423 = Replace Array Subset(array=w3349, new element=w3354, index (row)=w3350, index (col)=w3351) -> (w3348:string[][])
                        n1424 = local write "csv作成表_csv書込"(w3348) -> ()
                      }
                      frame True {
                        # "セルが空白だったらカウント1アップ"
                        n1425 = local read "空白列カウント 2"() -> (w3356:dbl)
                        n1426 = Add(x=w3356, y=1) -> (x+y=w3357:dbl)
                        n1427 = local write "空白列カウント 2"(w3357) -> ()
                      }
                    }
                  }
                }
              }
            }
          }
          frame #7 {
            # "④"
            # "csv書き込み\n値の書き込みが\nTrueだったらcsvファイル書き込み\nFalseだったら何もしない"
            n1428 = flat-sequence {
              frame #0 {
                n1429 = local read "保存ブール"() -> (w3358:bool)
                n1430 = case shown="FALSE" w3358 {
                  frame False {
                    n1431 = local read "CSV保存名"() -> (w3361:string)
                    n1432 = local read "書込CSV時間"() -> (w3359:string)
                    n1433 = local read "書込CSV日付"() -> (w3360:string)
                    n1434 = local read "CSV保存先"() -> (w3368:path)
                    n1435 = local read "csv作成表_csv書込"() -> (w3365:string[][])
                    n1436 = Concatenate Strings(w3361, "_", w3360, w3359, ".csv") -> (w3370:string)
                    n1437 = Build Path "パス作成"(base path=w3368, name or relative path=w3370) -> (appended path=w3371:path)
                    n1438 = One Button Dialog(message="CSV保存完了です", button name ("OK")="OK") -> ()  [unwired: 1 out]
                    n1439 = call-poly <vilib>:"Write Delimited Spreadsheet.vi"("file path (dialog if empty)"=w3371, "2D data"=w3365, "append to file? (new file:F)"=FALSE, "delimiter (\\t)"=",") -> ()  [unwired: 10 in, 2 out]
                  }
                  frame True {
                  }
                }
              }
            }
          }
          frame #8 {
            w3372 = 0
            n1440 = local read "csv作成表_csv書込_リセット用"() -> (w3374:string[][])
            n1441 = local read "csv作成表_リセット用"() -> (w3373:string[][])
            n1442 = local write "空白列カウント"(w3372) -> ()
            n1443 = local write "空白列カウント 2"(w3372) -> ()
            n1444 = local write "csv作成表_csv書込"(w3374) -> ()
            n1445 = local write "csv作成表"(w3373) -> ()
          }
        }
        n1446 = control-ref of="このVI"() -> (w3144:refnum<vi>)
        n1447 = property on="ペーン 2" class="Pane"("Origin"=w3146) -> ()  [unwired: 2 in, 2 out]
        n1448 = control-ref of="このVI"() -> (w3145:refnum<vi>)
        n1449 = Unbundle(w3146) -> ("Vertical"=w3143:i16)  [unwired: 1 out]
        n1450 = Unbundle(w3146) -> ()  [unwired: 2 out]
        n1451 = property on="ペーン 2" class="Pane"("Origin"=w3146) -> ()  [unwired: 2 in, 2 out]
        n1452 = call "メイン_装飾移動サブ.vi"("Y軸座標入力"=w3143, "VI入力"=w3144) -> ()  [unwired: 10 in]
        n1453 = call "メイン_装飾枠移動サブ.vi"("VI入力"=w3145) -> ()  [unwired: 11 in]
      }
      frame "値1クリア" {
        w3375 = ""
        # "③"
        # "②"
        # "①"
        # "複製したら\n①ケース名変更\n②③\nローカル変数変更\nのみでOK"
        # "項目別の値のクリアの為、項目配列の分だけ作成する"
        n1454 = local read "メイン設定_設定 1"() -> (w3379:T2)
        n1455 = Bundle By Name(cluster=w3379, "実測値(MAX)"=w3375, "実測値(MIN)"=w3375) -> (w3378:T2)
        n1456 = local write "メイン設定_設定 1"(w3378) -> ()
        n1457 = global write "測定値MAXMIN_G.vi" "測定値MAX/MINグローバル"(string[][] []) -> ()
      }
      frame "値2クリア" {
        w3380 = ""
        # "測定値MAX/MINグローバルの値を初期化する"
        # "②"
        # "①"
        # "複製したら変更する項目\n①②\nローカル変数\n\n変更のみでOK"
        # "項目別の値のクリアの為、項目配列の分だけ作成する"
        n1458 = local read "メイン設定_設定 2"() -> (w3384:T2)
        n1459 = Bundle By Name(cluster=w3384, "実測値(MAX)"=w3380, "実測値(MIN)"=w3380) -> (w3383:T2)
        n1460 = local write "メイン設定_設定 2"(w3383) -> ()
        n1461 = global write "測定値MAXMIN_G.vi" "測定値MAX/MINグローバル"(string[][] []) -> ()
      }
      frame "値3クリア" {
        w3385 = ""
        # "測定値MAX/MINグローバルの値を初期化する"
        # "②"
        # "①"
        # "複製したら変更する項目\n①②\nローカル変数\n\n変更のみでOK"
        # "項目別の値のクリアの為、項目配列の分だけ作成する"
        n1462 = local read "メイン設定_設定 3"() -> (w3389:T2)
        n1463 = Bundle By Name(cluster=w3389, "実測値(MAX)"=w3385, "実測値(MIN)"=w3385) -> (w3388:T2)
        n1464 = local write "メイン設定_設定 3"(w3388) -> ()
        n1465 = global write "測定値MAXMIN_G.vi" "測定値MAX/MINグローバル"(string[][] []) -> ()
      }
      frame "値4クリア" {
        w3390 = ""
        # "測定値MAX/MINグローバルの値を初期化する"
        # "②"
        # "①"
        # "複製したら変更する項目\n①②\nローカル変数\n\n変更のみでOK"
        # "項目別の値のクリアの為、項目配列の分だけ作成する"
        n1466 = local read "メイン設定_設定 4"() -> (w3394:T2)
        n1467 = Bundle By Name(cluster=w3394, "実測値(MAX)"=w3390, "実測値(MIN)"=w3390) -> (w3393:T2)
        n1468 = local write "メイン設定_設定 4"(w3393) -> ()
        n1469 = global write "測定値MAXMIN_G.vi" "測定値MAX/MINグローバル"(string[][] []) -> ()
      }
      frame "値5クリア" {
        w3395 = ""
        # "測定値MAX/MINグローバルの値を初期化する"
        # "②"
        # "①"
        # "複製したら変更する項目\n①②\nローカル変数\n\n変更のみでOK"
        # "項目別の値のクリアの為、項目配列の分だけ作成する"
        n1470 = local read "メイン設定_設定 5"() -> (w3399:T2)
        n1471 = Bundle By Name(cluster=w3399, "実測値(MAX)"=w3395, "実測値(MIN)"=w3395) -> (w3398:T2)
        n1472 = local write "メイン設定_設定 5"(w3398) -> ()
        n1473 = global write "測定値MAXMIN_G.vi" "測定値MAX/MINグローバル"(string[][] []) -> ()
      }
      frame "値6クリア" {
        w3400 = ""
        # "測定値MAX/MINグローバルの値を初期化する"
        # "②"
        # "①"
        # "複製したら変更する項目\n①②\nローカル変数\n\n変更のみでOK"
        # "項目別の値のクリアの為、項目配列の分だけ作成する"
